vi "DataAssignement.vi"(8 "ErrorIn (NoErr)":errorcluster caption="entrée d'erreur (pas d'erreur)", 11 "Experiment.lvclass":refnum<class "Experiment.lvclass">) -> (0 "ErrOut":errorcluster caption="sortie d'erreur", 3 "Experiment.lvclassOut":refnum<class "Experiment.lvclass">)   [LabVIEW 2019, in "BaseDevice.lvclass"]
uses:
  BaseDevice.lvclass
  Experiment Class/Experiment.lvclass
  BaseDevice.lvclass/BaseDevice.ctl
panel:
  in  "RemoveDat":bool
  in  "TargetData":u16(ring) caption="Target Assignment"
  out "Tableau 2":u32[][](array[numeric])
  out "Tableau":string[][](array[string])
  in  "AssignDat":bool
  in  "Stop":bool
  out "DeviceCtrls":T1(array[cluster])
  in  "SrcData":u16(ring) caption="Data Source" items=["Lambda", "InSlit", "OutSlit", "MiseAJour", "Grating", "Moving", "error in (no error)", "error out", "Triax320.lvclass", "Triax320.lvclass Out", "Init Program", "Stop", "GrooveRatio"]
  in  "SrcInstr":u16(ring) caption="Source Instrument" items=["Triax320", "Tools", "SympCCD"]
  in  "TargetInstr":u16(ring) caption="Target Instrument" items=["Triax320", "Tools", "SympCCD"]
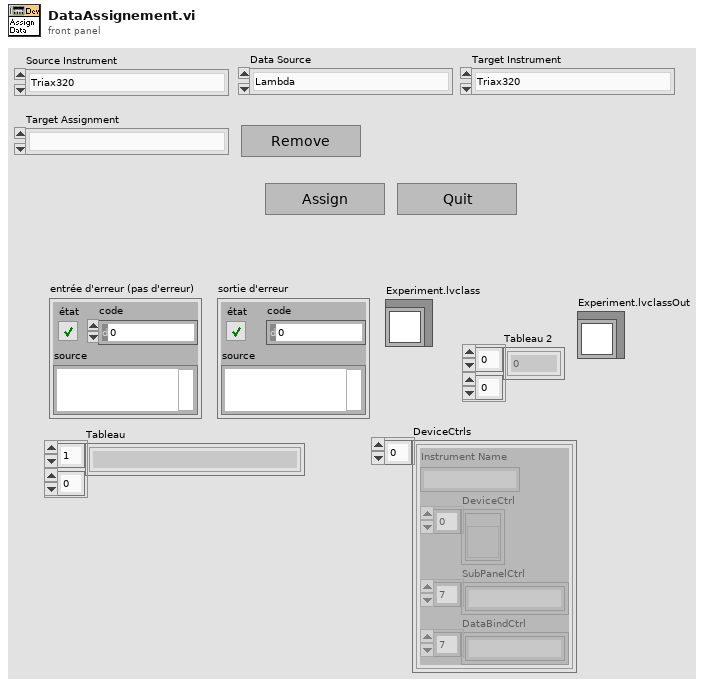
[diagram p1: front panel]
types:
  T1 = cluster{"Instrument Name":string, "DeviceCtrl":refnum<vi>[], "SubPanelCtrl":string[], "DataBindCtrl":string[]}[]
  T2 = cluster{"Message":string, "Data":variant, "Code":i32}
  T3 = cluster{"Instrument Name":string, "DeviceCtrl":refnum<vi>[], "SubPanelCtrl":string[], "DataBindCtrl":string[]}
  T4 = cluster{"InstrumentName":string, "DeviceCtrl":refnum<vi>[], "SubPanelCtrl":string[], "DataBindCtrl":string[]}
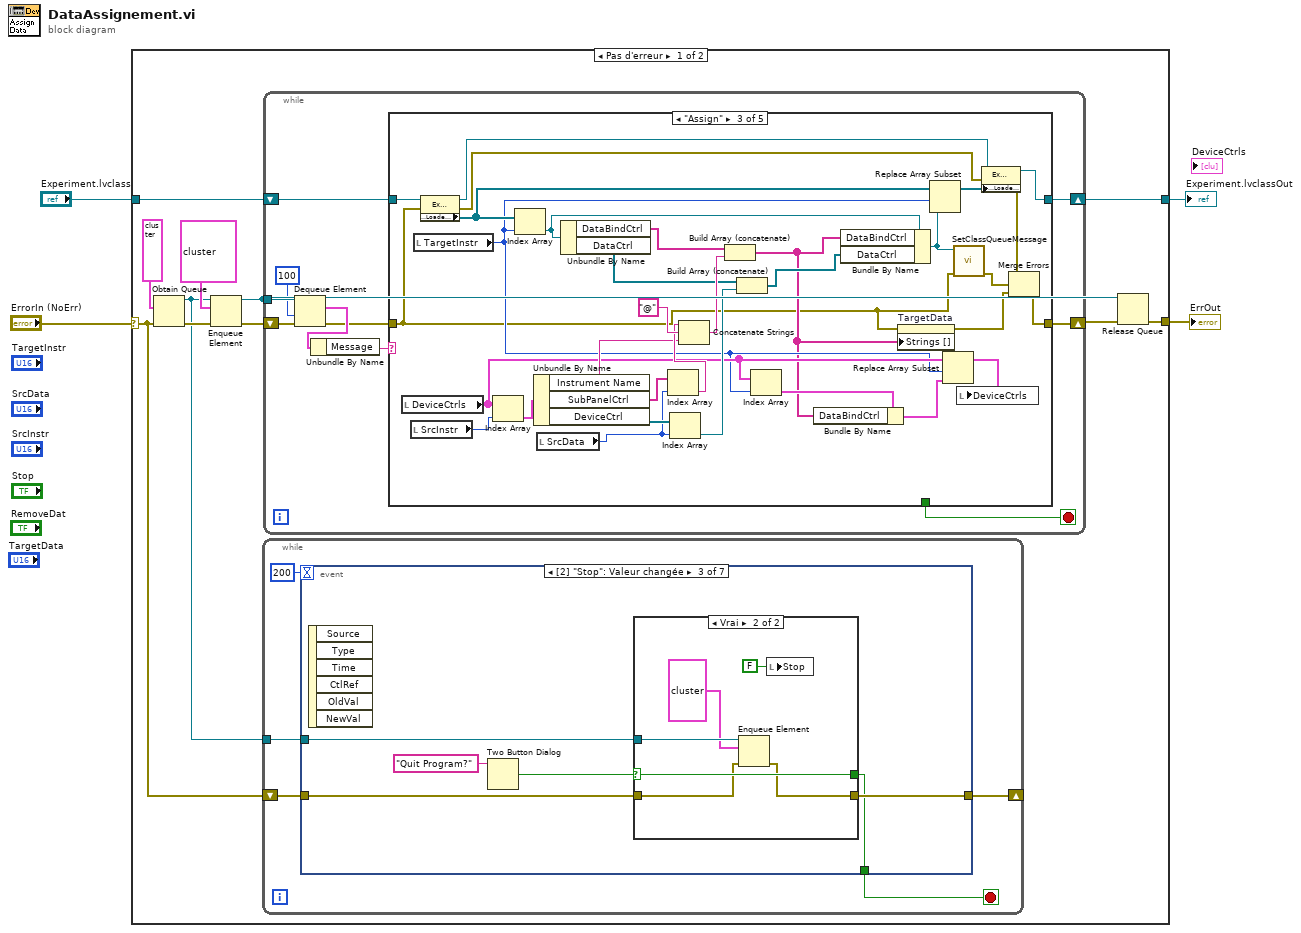
[diagram p0: block diagram]
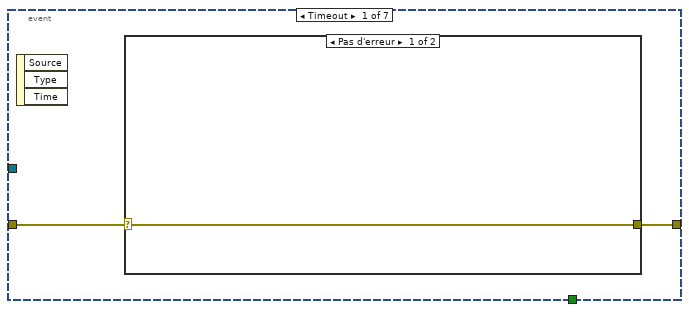
[diagram p2: hidden frame]
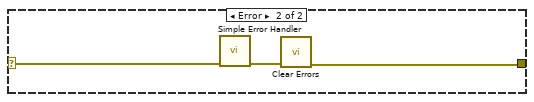
[diagram p3: hidden frame]
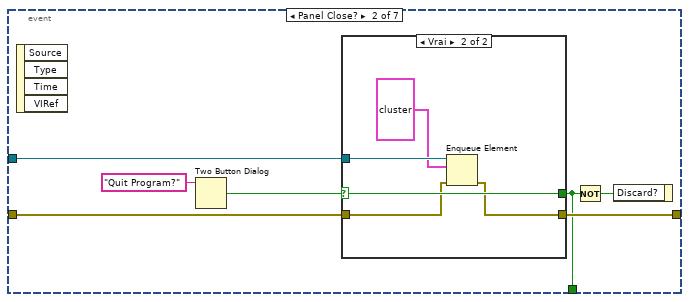
[diagram p4: hidden frame]
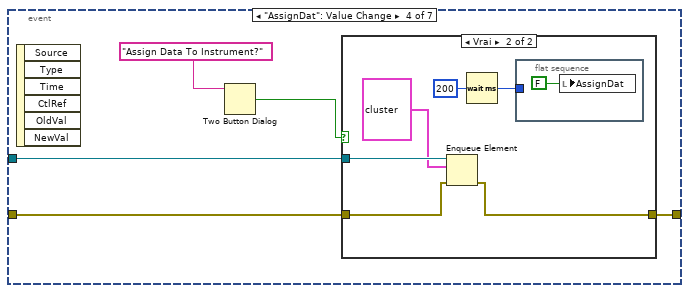
[diagram p7: hidden frame]
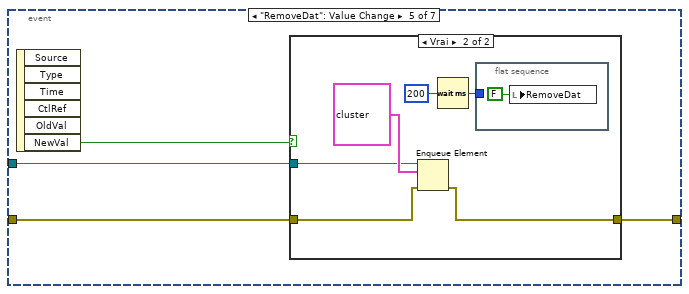
[diagram p9: hidden frame]
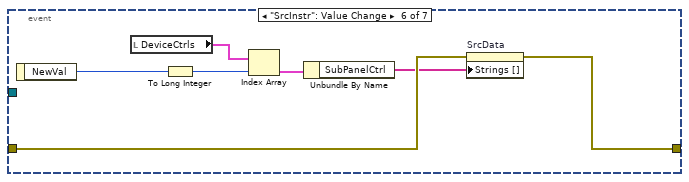
[diagram p11: hidden frame]
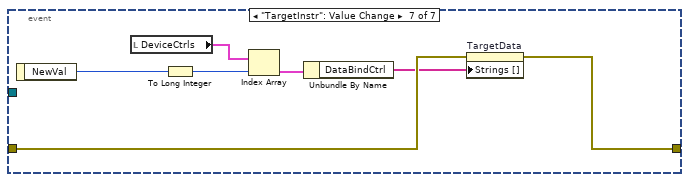
[diagram p12: hidden frame]
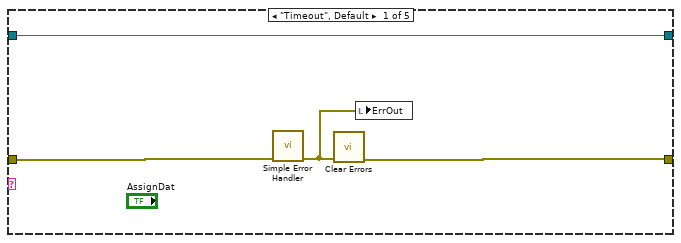
[diagram p13: hidden frame]
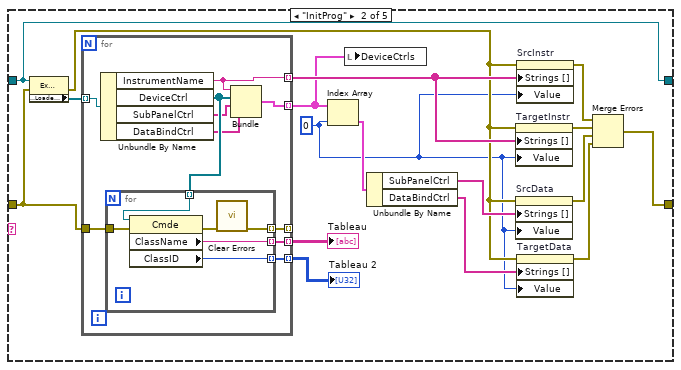
[diagram p14: hidden frame]
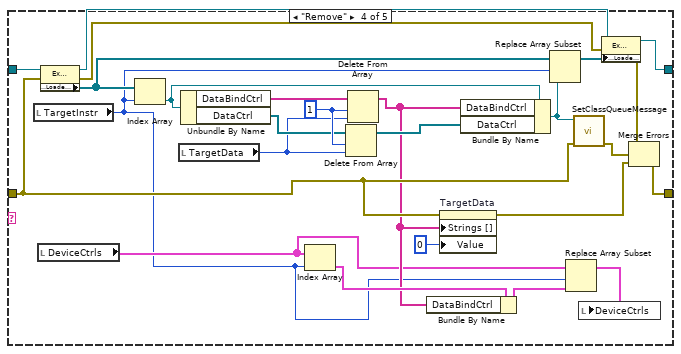
[diagram p15: hidden frame]
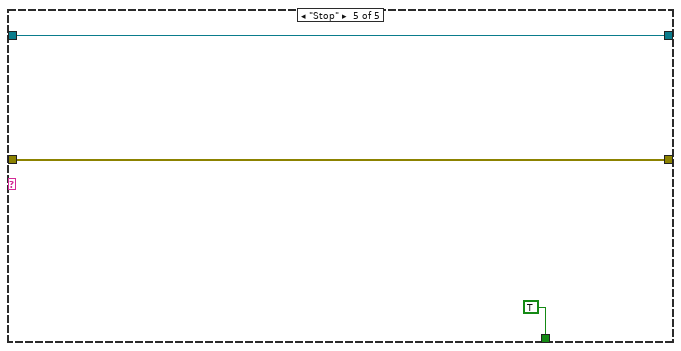
[diagram p16: hidden frame]
diagram:
  n1 = case shown="Pas d'erreur" "ErrorIn (NoErr)" {
    selector: "ErrorIn (NoErr)" -> [w10 w201]
    tunnel: "Experiment.lvclass" -> [w15 w202]
    tunnel: [w7 w202] -> w2
    tunnel: [w5 w201] -> w1
    frame No Error {
      n2 = Obtain Queue(element data type=T2 {"Message"="", "Data"=variant, "Code"=0} ("élément"), error in (no error)=w10) -> (queue out=w9:refnum<queue>, error out=w13:errorcluster)  [unwired: 3 in, 1 out]
      n3 = Enqueue Element(queue=w9, element=T2 {"Message"="InitProg", "Data"=variant, "Code"=0} ("élément"), error in (no error)=w13) -> (queue out=w8:refnum<queue>, error out=w12:errorcluster)  [unwired: 1 in, 1 out]
      n4 = while {
        tunnel: w9 -> [w18]
        shift-right: [w17] -> _
        shift-left: w10 -> [w19]
        stop <- w16 stop-if-true
        n5 = event shown="[2] \"Stop\": Valeur changée" {
          selector: _ -> [_ _ _ _ _ _ _]
          dyn-events: _ -> [_ _ _ _ _ _ _]
          timeout: 200 -> [_ _ _ _ _ _ _]
          tunnel: w19 -> [w22 w29 w43 w58 w69 w82 w89]
          tunnel: w18 -> [_ w33 w46 w59 w70 _ _]
          tunnel: [w21 w28 w42 w57 w68 w80 w87] -> w17
          tunnel: [_ w27 w41 _ _ _ _] -> w16
          event Timeout {
            n6 = event-data() -> ()  [unwired: 1 in, 3 out]
            n7 = case shown="Pas d'erreur" w22 {
              selector: w22 -> [w23 w26]
              tunnel: [w23 w24] -> w21
              frame No Error {
              }
              frame Error {
                n8 = call <vilib>:"Simple Error Handler.vi"("error in (no error)"=w26) -> ("error out"=w25:errorcluster)  [unwired: 4 in, 4 out]
                n9 = call <vilib>:"Clear Errors.vi"("error in (no error)"=w25) -> ("error out"=w24:errorcluster)  [unwired: 5 in, 1 out]
              }
            }
          }
          event Panel Close? {
            n10 = event-data() -> ()  [unwired: 1 in, 4 out]
            n11 = Two Button Dialog(message="Quit Program?") -> (T button?=w32:bool)  [unwired: 2 in]
            n12 = case shown="Vrai" w32 {
              selector: w32 -> [w35 w38]
              tunnel: w33 -> [_ w40]
              tunnel: [w35 w38] -> w27
              tunnel: w29 -> [w34 w37]
              tunnel: [w34 w36] -> w28
              frame False {
              }
              frame True {
                n13 = Enqueue Element(queue=w40, element=T2 {"Message"="Stop", "Data"=variant, "Code"=0} ("élément"), error in (no error)=w37) -> (error out=w36:errorcluster)  [unwired: 1 in, 2 out]
              }
            }
            n14 = Not(x=w27) -> (.not. x?=w30:bool)
            n15 = event-data("Discard?"=w30) -> ()  [unwired: 1 in, 1 out]
          }
          event "Stop": Value Change {
            n16 = event-data() -> ()  [unwired: 1 in, 6 out]
            n17 = Two Button Dialog(message="Quit Program?") -> (T button?=w45:bool)  [unwired: 2 in]
            n18 = case shown="Vrai" w45 {
              selector: w45 -> [w48 w52]
              tunnel: w46 -> [_ w54]
              tunnel: [w48 w52] -> w41
              tunnel: w43 -> [w47 w51]
              tunnel: [w47 w50] -> w42
              frame False {
              }
              frame True {
                n19 = Enqueue Element(queue=w54, element=T2 {"Message"="Stop", "Data"=variant, "Code"=0} ("élément"), error in (no error)=w51) -> (error out=w50:errorcluster)  [unwired: 1 in, 2 out]
                n20 = local write "Stop"(FALSE ("Stop")) -> ()
              }
            }
          }
          event "AssignDat": Value Change {
            n21 = event-data() -> ()  [unwired: 1 in, 6 out]
            n22 = Two Button Dialog(message="Assign Data To Instrument?") -> (T button?=w55:bool)  [unwired: 2 in]
            n23 = case shown="Vrai" w55 {
              tunnel: w59 -> [_ w66]
              tunnel: w58 -> [w60 w64]
              tunnel: [w60 w63] -> w57
              frame False {
              }
              frame True {
                n24 = Enqueue Element(queue=w66, element=T2 {"Message"="Assign", "Data"=variant, "Code"=0} ("élément"), error in (no error)=w64) -> (error out=w63:errorcluster)  [unwired: 1 in, 2 out]
                n25 = Wait (ms)(milliseconds to wait=u32 200 ("attente (ms)")) -> (millisecond timer value=w61:u32)
                n26 = flat-sequence {
                  tunnel: w61 -> [_]
                  frame #0 {
                    n27 = local write "AssignDat"(FALSE ("Stop")) -> ()
                  }
                }
              }
            }
          }
          event "RemoveDat": Value Change {
            n28 = event-data() -> ("NewVal"=w71:bool)  [unwired: 1 in, 5 out]
            n29 = case shown="Vrai" w71 {
              tunnel: w70 -> [_ w76]
              tunnel: w69 -> [w72 w75]
              tunnel: [w72 w73] -> w68
              frame False {
              }
              frame True {
                n30 = Enqueue Element(queue=w76, element=T2 {"Message"="Remove", "Data"=variant, "Code"=0} ("élément"), error in (no error)=w75) -> (error out=w73:errorcluster)  [unwired: 1 in, 2 out]
                n31 = Wait (ms)(milliseconds to wait=u32 200 ("attente (ms)")) -> (millisecond timer value=w74:u32)
                n32 = flat-sequence {
                  tunnel: w74 -> [_]
                  frame #0 {
                    n33 = local write "RemoveDat"(FALSE ("RemoveDat")) -> ()
                  }
                }
              }
            }
          }
          event "SrcInstr": Value Change {
            n34 = event-data() -> ("NewVal"=w86:u16)  [unwired: 1 in]
            n35 = local read "DeviceCtrls"() -> (w85:T1)
            n36 = To Long Integer(number=w86) -> (32bit integer=w84:i32)
            n37 = Index Array(array=w85, index=w84) -> (element=w83:T3)
            n38 = Unbundle By Name(w83) -> ("SubPanelCtrl"=w81:string[])
            n39 = property on="SrcData" class="MDér (strict)"(error in=w82, "Strings []"=w81) -> (error out=w80:errorcluster)  [unwired: 1 in, 1 out]
          }
          event "TargetInstr": Value Change {
            n40 = event-data() -> ("NewVal"=w93:u16)  [unwired: 1 in]
            n41 = local read "DeviceCtrls"() -> (w92:T1)
            n42 = To Long Integer(number=w93) -> (32bit integer=w91:i32)
            n43 = Index Array(array=w92, index=w91) -> (element=w90:T3)
            n44 = Unbundle By Name(w90) -> ("DataBindCtrl"=w88:string[])
            n45 = property on="TargetData" class="MDér (strict)"(error in=w89, "Strings []"=w88) -> (error out=w87:errorcluster)  [unwired: 1 in, 1 out]
          }
        }
      }
      n46 = while {
        shift-right: [w96] -> w6
        shift-left: w12 -> [w103]
        shift-right: [w97] -> w7
        shift-left: w15 -> [w100]
        tunnel: w8 -> [w98]
        stop <- w95 stop-if-true
        n47 = Dequeue Element(queue=w98, timeout in ms (-1)=100 ("timeout en ms (-1)"), error in (no error)=w103) -> (element=w102:T2, error out=w99:errorcluster)  [unwired: 2 out]
        n48 = Unbundle By Name(w102) -> ("Message"=w101:string)
        n49 = case shown="\"Assign\"" w101 {
          tunnel: w100 -> [w107 w121 w172 w197 w200]
          tunnel: w99 -> [w106 w112 w142 w182 w199]
          tunnel: [w107 w121 w163 w193 w200] -> w97
          tunnel: [w105 w119 w150 w188 w199] -> w96
          tunnel: [_ _ _ _ TRUE ("Stop")] -> w95
          frame "Timeout", Default {
            n50 = call <vilib>:"Simple Error Handler.vi"("error in (no error)"=w106) -> ("error out"=w104:errorcluster)  [unwired: 4 in, 4 out]
            n51 = call <vilib>:"Clear Errors.vi"("error in (no error)"=w104) -> ("error out"=w105:errorcluster)  [unwired: 5 in, 1 out]
            n52 = local write "ErrOut"(w104) -> ()
          }
          frame "InitProg" {
            w108 = 0 ("indice (ligne)")
            n53 = property class="Experiment.lvclass"(reference=w121, error in=w112) -> (error out=w110:errorcluster, "Accessor:LoadedInst"=w124:refnum<class "BaseDevice.lvclass">[])  [unwired: 1 out]
            n54 = for {
              tunnel: w124 -> [w134] mode=indexing
              tunnel: [w130] -> w116 mode=indexing
              tunnel: [w133] -> w115 mode=indexing
              tunnel: [w132] -> w113 mode=indexing
              tunnel: [w131] -> w114 mode=indexing
              tunnel: w112 -> [w129]
              tunnel: [w128] -> _ mode=indexing
              n55 = Unbundle By Name(w134) -> ("InstrumentName"=w130:string, "DeviceCtrl"=w127:refnum<vi>[], "SubPanelCtrl"=w126:string[], "DataBindCtrl"=w125:string[])
              n56 = for {
                tunnel: w127 -> [w140] mode=indexing
                tunnel: [w139] -> w132 mode=indexing
                tunnel: [w138] -> w131 mode=indexing
                tunnel: w129 -> [w137]
                tunnel: [w135] -> w128 mode=indexing
                n57 = property class="Cmde"(reference=w140, error in=w137) -> (error out=w136:errorcluster, "ClassName"=w138:string, "ClassID"=w139:u32)  [unwired: 1 out]
                n58 = call <vilib>:"Clear Errors.vi"("error in (no error)"=w136) -> ("error out"=w135:errorcluster)  [unwired: 5 in, 1 out]
              }
              n59 = Bundle("InstrumentName"=w130, "DeviceCtrl"=w127, "SubPanelCtrl"=w126, "DataBindCtrl"=w125) -> (w133:T4)  [unwired: 1 in]
            }
            "Tableau" <- w114
            "Tableau 2" <- w113
            n60 = Index Array(array=w115, index=w108) -> (element=w123:T4)
            n61 = local write "DeviceCtrls"(w115) -> ()
            n62 = Unbundle By Name(w123) -> ("SubPanelCtrl"=w122:string[], "DataBindCtrl"=w111:string[])
            n63 = property on="TargetInstr" class="MDér (strict)"(error in=w110, "Strings []"=w116, "Value"=w108) -> (error out=w117:errorcluster)  [unwired: 1 in, 1 out]
            n64 = property on="SrcData" class="MDér (strict)"(error in=w110, "Strings []"=w122, "Value"=w108) -> (error out=w118:errorcluster)  [unwired: 1 in, 1 out]
            n65 = property on="SrcInstr" class="MDér (strict)"(error in=w110, "Strings []"=w116, "Value"=w108) -> (error out=w120:errorcluster)  [unwired: 1 in, 1 out]
            n66 = property on="TargetData" class="MDér (strict)"(error in=w110, "Strings []"=w111, "Value"=w108) -> (error out=w109:errorcluster)  [unwired: 1 in, 1 out]
            n67 = Merge Errors(w120, w117, w118, w109) -> (w119:errorcluster)
          }
          frame "Assign" {
            n68 = local read "DeviceCtrls"() -> (w147:T1)
            n69 = local read "SrcInstr"() -> (w171:u16)
            n70 = local read "TargetInstr"() -> (w146:u16)
            n71 = property class="Experiment.lvclass"(reference=w172, error in=w142) -> (reference out=w164:refnum<class "Experiment.lvclass">, error out=w153:errorcluster, "Accessor:LoadedInst"=w166:refnum<class "BaseDevice.lvclass">[])
            n72 = Index Array(array=w147, index=w171) -> (element=w170:T3)
            n73 = Index Array(array=w166, index=w146) -> (element=w157:refnum<class "BaseDevice.lvclass">)
            n74 = Unbundle By Name(w170) -> ("Instrument Name"=w158:string, "SubPanelCtrl"=w162:string[], "DeviceCtrl"=w169:refnum<vi>[])
            n75 = local read "SrcData"() -> (w168:u16)
            n76 = Unbundle By Name(w157) -> ("DataBindCtrl"=w156:string[], "DataCtrl"=w155:refnum<vi>[])
            n77 = Index Array(array=w162, index=w168) -> (element=w159:string)
            n78 = Index Array(array=w169, index=w168) -> (element=w167:refnum<vi>)
            n79 = Concatenate Strings(w159, "@" ("chaîne"), w158) -> (w160:string)
            n80 = Build Array (concatenate)(w156, w160) -> (w143:string[])
            n81 = Build Array (concatenate)(w155, w167) -> (w154:refnum<vi>[])
            n82 = Index Array(array=w147, index=w146) -> (element=w148:T3)
            n83 = Bundle By Name(cluster=w148, "DataBindCtrl"=w143) -> (w144:T3)
            n84 = Bundle By Name(cluster=w157, "DataBindCtrl"=w143, "DataCtrl"=w154) -> (w152:refnum<class "BaseDevice.lvclass">)
            n85 = property on="TargetData" class="MDér (strict)"(error in=w142, "Strings []"=w143) -> (error out=w141:errorcluster)  [unwired: 1 in, 1 out]
            n86 = Replace Array Subset(array=w166, new element=w152, index=w146) -> (w165:refnum<class "BaseDevice.lvclass">[])
            n87 = Replace Array Subset(array=w147, new element=w144, index=w146) -> (w145:T1)
            n88 = call-dynamic "SetClassQueueMessage.vi"("ErrorIn(No Error)"=w142, "BaseDevice.lvclass"=w152) -> ("sortie d'erreur"=w149:errorcluster)  [unwired: 8 in, 1 out]
            n89 = local write "DeviceCtrls"(w145) -> ()
            n90 = property class="Experiment.lvclass"(reference=w164, error in=w153, "Accessor:LoadedInst"=w165) -> (reference out=w163:refnum<class "Experiment.lvclass">, error out=w151:errorcluster)
            n91 = Merge Errors(w151, w149, w141) -> (w150:errorcluster)
          }
          frame "Remove" {
            w185 = 1 ("longueur")
            n92 = local read "TargetInstr"() -> (w176:u16)
            n93 = local read "DeviceCtrls"() -> (w177:T1)
            n94 = property class="Experiment.lvclass"(reference=w197, error in=w182) -> (reference out=w194:refnum<class "Experiment.lvclass">, error out=w191:errorcluster, "Accessor:LoadedInst"=w196:refnum<class "BaseDevice.lvclass">[])
            n95 = Index Array(array=w196, index=w176) -> (element=w192:refnum<class "BaseDevice.lvclass">)
            n96 = local read "TargetData"() -> (w174:u16)
            n97 = Unbundle By Name(w192) -> ("DataBindCtrl"=w186:string[], "DataCtrl"=w183:refnum<vi>[])
            n98 = Index Array(array=w177, index=w176) -> (element=w180:T3)
            n99 = Delete From Array(array=w183, length=w185, index=w174) -> (array with subset deleted=w184:refnum<vi>[])  [unwired: 1 out]
            n100 = Delete From Array(array=w186, length=w185, index=w174) -> (array with subset deleted=w178:string[])  [unwired: 1 out]
            n101 = Bundle By Name(cluster=w180, "DataBindCtrl"=w178) -> (w179:T3)
            n102 = property on="TargetData" class="MDér (strict)"(error in=w182, "Strings []"=w178, "Value"=0) -> (error out=w181:errorcluster)  [unwired: 1 in, 1 out]
            n103 = Bundle By Name(cluster=w192, "DataBindCtrl"=w178, "DataCtrl"=w184) -> (w190:refnum<class "BaseDevice.lvclass">)
            n104 = Replace Array Subset(array=w196, new element=w190, index=w176) -> (w195:refnum<class "BaseDevice.lvclass">[])
            n105 = Replace Array Subset(array=w177, new element=w179, index=w176) -> (w175:T1)
            n106 = call-dynamic "SetClassQueueMessage.vi"("ErrorIn(No Error)"=w182, "BaseDevice.lvclass"=w190) -> ("sortie d'erreur"=w187:errorcluster)  [unwired: 8 in, 1 out]
            n107 = local write "DeviceCtrls"(w175) -> ()
            n108 = property class="Experiment.lvclass"(reference=w194, error in=w191, "Accessor:LoadedInst"=w195) -> (reference out=w193:refnum<class "Experiment.lvclass">, error out=w189:errorcluster)
            n109 = Merge Errors(w189, w187, w181) -> (w188:errorcluster)
          }
          frame "Stop" {
          }
        }
      }
      n110 = Release Queue(queue=w8, error in (no error)=w6) -> (error out=w5:errorcluster)  [unwired: 1 in, 2 out]
    }
    frame Error {
    }
  }
  "Experiment.lvclassOut" <- w2
  "ErrOut" <- w1
